vi "arraytextring.vi"(1 "Array In":i32[](array[ring]) items=["One"=1, "Two"=2, "Three"=3, "Four"=4, "Five"=5, "Six"=6, "Seven"=7, "Eight"=8, "Nine"=9, "Ten"=10, "Eleven"=11, "Twelve"=12, "Thirteen"=13, "Fourteen"=14, "Fifteen"=15]) -> (0 "Array Out":i32[](array[ring]) items=["One"=1, "Two"=2, "Three"=3, "Four"=4, "Five"=5, "Six"=6, "Seven"=7, "Eight"=8, "Nine"=9, "Ten"=10, "Eleven"=11, "Twelve"=12, "Thirteen"=13, "Fourteen"=14, "Fifteen"=15])   [LabVIEW 2011]
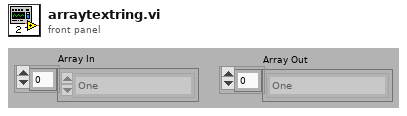
[diagram p1: front panel]
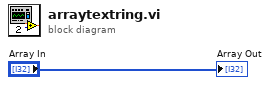
[diagram p0: block diagram]
diagram:
  "Array Out" <- "Array In"
